vi "CheckonTheInputData_171213.vi"(11 "InputArray":sgl[][](array[numeric])) -> (3 "OutputArray":sgl[](array[numeric]))   [LabVIEW 2018]
panel:
  out "OldArray":sgl[](array[numeric])
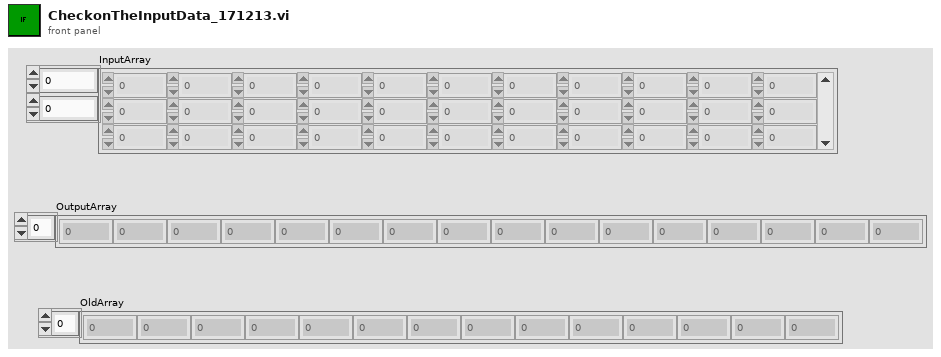
[diagram p1: front panel]
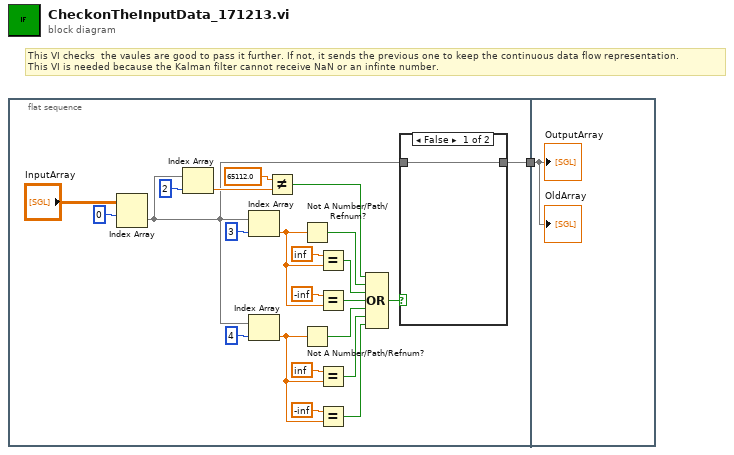
[diagram p0: block diagram]
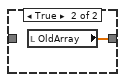
[diagram p2: hidden frame]
diagram:
  # "This VI checks  the vaules are good to pass it further. If not, it sends the previous one to keep the continuous data flow representation.\nThis VI is needed because the Kalman filter cannot receive NaN or an infinte number."
  n1 = flat-sequence {
    tunnel: [w2] -> w1
    tunnel: w1 -> [w27]
    frame #0 {
      n2 = Index Array(array="InputArray", index (row)=0) -> (element=w6:sgl[])  [unwired: 1 in]
      n3 = Index Array(array=w6, index=2 ("disabled index (col)")) -> (element=w23:sgl)
      n4 = Index Array(array=w6, index=3 ("disabled index (col)")) -> (element=w20:sgl)
      n5 = Index Array(array=w6, index=4 ("disabled index (col)")) -> (element=w13:sgl)
      n6 = Not Equal?(x=65112.0, y=w23) -> (x != y?=w19:bool)
      n7 = Not A Number/Path/Refnum?(number/path/refnum=w20) -> (NaN/Path/Refnum?=w18:bool)
      n8 = Not A Number/Path/Refnum?(number/path/refnum=w13) -> (NaN/Path/Refnum?=w12:bool)
      n9 = Equal?(x=inf, y=w20) -> (x = y?=w17:bool)
      n10 = Equal?(x=-inf, y=w20) -> (x = y?=w16:bool)
      n11 = Equal?(x=inf, y=w13) -> (x = y?=w11:bool)
      n12 = Equal?(x=-inf, y=w13) -> (x = y?=w10:bool)
      n13 = Compound Arithmetic op=OR(w19, w18, w17, w16, w12, w11, w10) -> (w9:bool)
      n14 = case shown="False" w9 {
        tunnel: w6 -> [w25 _]
        tunnel: [w25 w26] -> w2
        frame False {
        }
        frame True {
          n15 = local read "OldArray"() -> (w26:sgl[])
        }
      }
    }
    frame #1 {
      "OutputArray" <- w27
      "OldArray" <- w27
    }
  }
